vi "Check Compatibility for CSM.vi"(6 "force check(F)":bool, 8 "Error in":errorcluster caption="Error in (no error)") -> (0 "Error out":errorcluster, 3 "Compactible":bool)   [LabVIEW 2017, in "Communicable State Machine.lvlib"]
uses:
  Communicable State Machine.lvlib
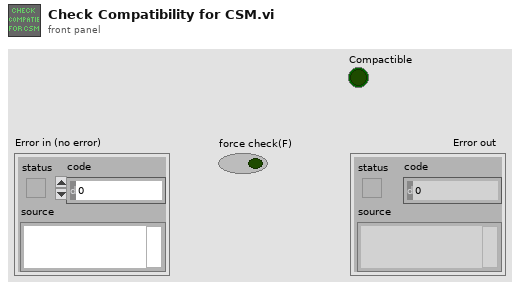
[diagram p1: front panel]
types:
  T1 = cluster{"Major":u16, "Minor":u16, "Fix":u16, "Build":u16}
  T2 = cluster{"Major":bool, "Minor":bool, "Fix":bool, "Build":bool}
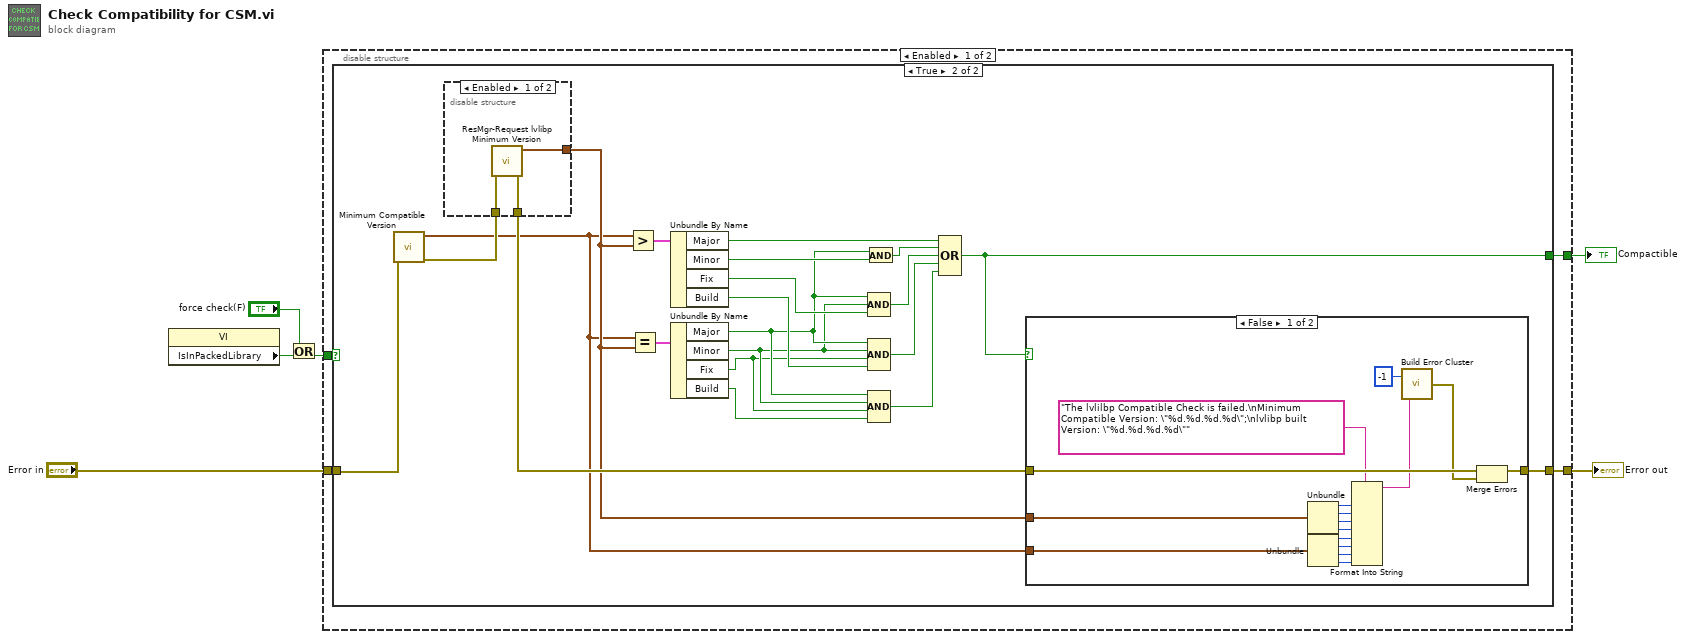
[diagram p0: block diagram]
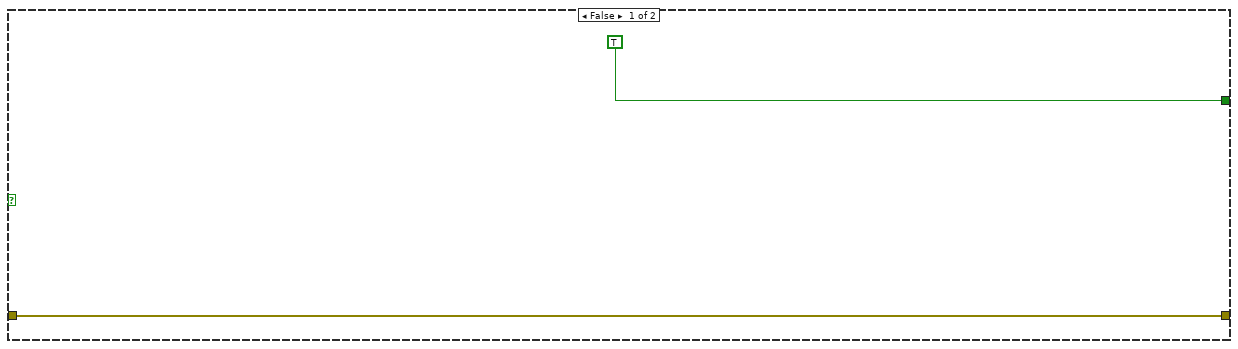
[diagram p2: hidden frame]
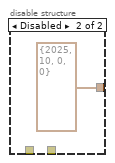
[diagram p3: hidden frame]
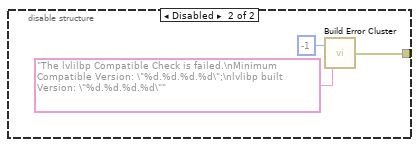
[diagram p5: hidden frame]
diagram:
  n1 = property class="VI"() -> ("IsInPackedLibrary"=w4:bool)  [unwired: 2 in, 2 out]
  n2 = Or(x="force check(F)", y=w4) -> (x .or. y?=w2:bool)
  n3 = disable-structure shown="Enabled" {
    disable-tunnel: [w10 w55] -> w6
    disable-tunnel: "Error in" -> [w9 _]
    disable-tunnel: [w8 _] -> w3
    disable-tunnel: w2 -> [w7 _]
    frame Enabled {
      n4 = case shown="True" w7 {
        tunnel: [w12 w16] -> w10
        tunnel: w9 -> [w12 w33]
        tunnel: [TRUE w13] -> w8
        frame False {
        }
        frame True {
          n5 = call "Minimum Compatible Version.vi"("Error in"=w33) -> ("Error out"=w32:errorcluster, "Min-Compatible Version"=w14:T1)  [unwired: 9 in]
          n6 = disable-structure shown="Enabled" {
            disable-tunnel: w32 -> [w36 _]
            disable-tunnel: [w35 _] -> w31
            disable-tunnel: [w34 T1 {"Major"=2025, "Minor"=10, "Fix"=0, "Build"=0} ("CSM Version")] -> w15
            frame Enabled {
              n7 = call "ResMgr-Request lvlibp Minimum Version.vi"("Error In"=w36) -> ("error out"=w35:errorcluster, "CSM Version"=w34:T1)  [unwired: 9 in]
            }
            frame Disabled {
            }
          }
          n8 = Greater?(x=w14, y=w15) -> (0:w30:T2)
          n9 = Equal?(x=w14, y=w15) -> (x = y?=w29:T2)
          n10 = Unbundle By Name(w30) -> ("Major"=w28:bool, "Minor"=w27:bool, "Fix"=w25:bool, "Build"=w23:bool)
          n11 = Unbundle By Name(w29) -> ("Major"=w22:bool, "Minor"=w21:bool, "Fix"=w20:bool, "Build"=w19:bool)
          n12 = And(x=w22, y=w27) -> (x .and. y?=w26:bool)
          n13 = Compound Arithmetic op=AND(w22, w21, w25) -> (w24:bool)
          n14 = Compound Arithmetic op=AND(w22, w21, w20, w23) -> (w18:bool)
          n15 = Compound Arithmetic op=AND(w22, w21, w20, w19) -> (w17:bool)
          n16 = Compound Arithmetic op=OR(w28, w26, w24, w18, w17) -> (w13:bool)
          n17 = case shown="False" w13 {
            tunnel: w31 -> [w53 w54]
            tunnel: [w51 w54] -> w16
            tunnel: w15 -> [w47 _]
            tunnel: w14 -> [w46 _]
            frame False {
              n18 = Unbundle(w47) -> ("Major"=w45:u16, "Minor"=w44:u16, "Fix"=w43:u16, "Build"=w42:u16)
              n19 = Unbundle(w46) -> ("Major"=w41:u16, "Minor"=w40:u16, "Fix"=w39:u16, "Build"=w38:u16)
              n20 = Format Into String(format string="The lvlilbp Compatible Check is failed.\nMinimum Compatible Version: \"%d.%d.%d.%d\";\nlvlibp built Version: \"%d.%d.%d.%d\"" ("String to Prepend to Source (\"\")"), w45, w44, w43, w42, w41, w40, w39, w38) -> (resulting string=w48:string)  [unwired: 2 in, 1 out]
              n21 = call "Build Error Cluster.vi"("String to Prepend to Source (\"\")"=w48, "Code"=-1) -> ("error out"=w50:errorcluster)
              n22 = Merge Errors(w53, w50) -> (w51:errorcluster)
            }
            frame True {
            }
          }
        }
      }
    }
    frame Disabled {
      n23 = call "Build Error Cluster.vi"("String to Prepend to Source (\"\")"="The lvlilbp Compatible Check is failed.\nMinimum Compatible Version: \"%d.%d.%d.%d\";\nlvlibp built Version: \"%d.%d.%d.%d\"" ("String to Prepend to Source (\"\")"), "Code"=-1) -> ("error out"=w55:errorcluster)
    }
  }
  "Error out" <- w6
  "Compactible" <- w3
